vi "IntegerSynByteArray2.vi"(6 "Mode":T2(ring), 8 "Clock multiplier":u32=64, 9 "Local Oscillator (IF,f2)":u32, 10 "f (f1)":u32, 11 "Phase (degrees)":dbl=90.0) -> (1 "Actual ratios":T1 {"Clock" format="%_20p"; "F2" format="%_20p"; "F1" format="%_20p"; "Clock/F2" format="%_20g"; "Clock/F1" format="%_20g"}, 3 "output array":u8[](array[numeric]) format="%08b")   [LabVIEW 2015]
uses:
  Actual settings.ctl
panel:
  out "Clock":i32
  out "phase":u8 format="%08b"
  # "Heterodyne"
  # "IOtech      Synth           NatInstBrd\n              function          J7          P3                   P1\n              syn1 w clk       A0           3             P0.0  1\n              syn1 D7           A1           5             P0.1  3\n              syn2 w clk       A2           7             PO.2  5\n              syn2 D7           A3           9             PO.3  7\n              syn3 w clk       A4           4             PO.4  9\n              syn3 D7           A5           6             P0.5   11\n              syn1,2 FQ_UD  A6           8             PO.6   13\n              syn3 FQ_UD     A7          10            PO.7   15\n\n              Reset 1,2,3     B4          14             PFI3   23\n\n              SCLK              B0           13            PFI 0  17\n              SYNC              B1           15            PFI 1  19\n              DIN                B2           17             PFI 2  21"
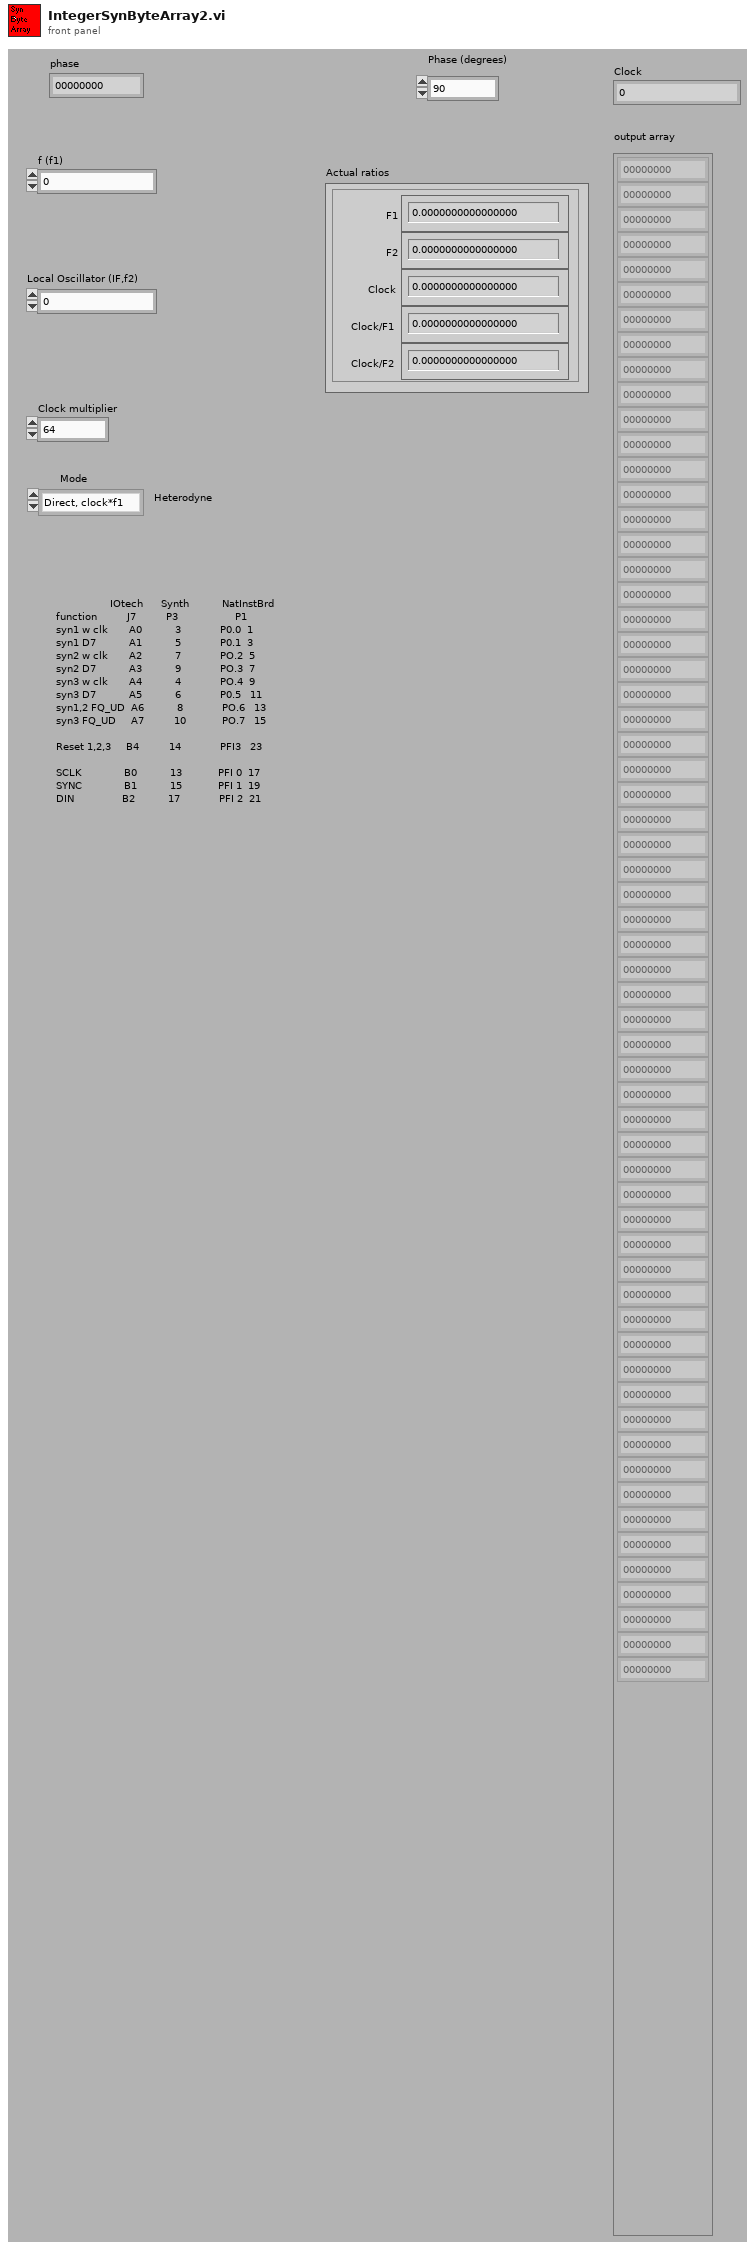
[diagram p1: front panel]
types:
  T1 = typedef "Actual settings.ctl" = cluster{"Clock/F1":ext, "Clock/F2":ext, "F1":ext, "F2":ext, "Clock":ext}
  T2 = enum16{"Direct, clock*f1", "Direct, clock*f2", "Heterodyne"}
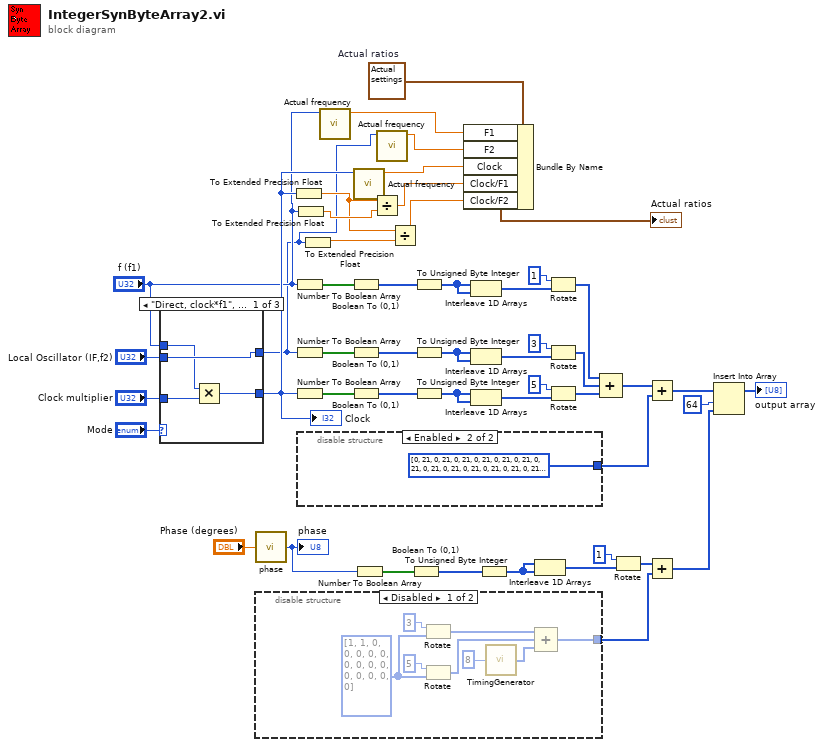
[diagram p0: block diagram]
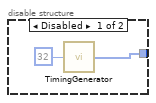
[diagram p2: hidden frame]
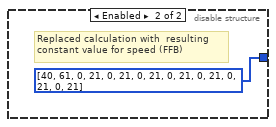
[diagram p3: hidden frame]
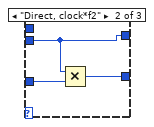
[diagram p4: hidden frame]
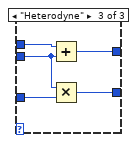
[diagram p5: hidden frame]
diagram:
  w7 = T1 {"Clock/F1"=64.0, "Clock/F2"=39.999998690327429603, "F1"=0.0, "F2"=0.0, "Clock"=0.0}  # Actual ratios
  n1 = case shown="\"Direct, clock*f1\", Default" "Mode" {
    tunnel: "Local Oscillator (IF,f2)" -> [w51 w54 w59]
    tunnel: [w53 w56 w61] -> w6
    tunnel: "Clock multiplier" -> [w52 w55 w60]
    tunnel: [w51 w54 w57] -> w2
    tunnel: "f (f1)" -> [w50 _ w58]
    frame "Direct, clock*f1", Default {
      n2 = Multiply(x=w50, y=w52) -> (x*y=w53:u32)
    }
    frame "Direct, clock*f2" {
      n3 = Multiply(x=w54, y=w55) -> (x*y=w56:u32)
    }
    frame "Heterodyne" {
      n4 = Add(x=w58, y=w59) -> (x+y=w57:u32)
      n5 = Multiply(x=w59, y=w60) -> (x*y=w61:u32)
    }
  }
  "Clock" <- w6
  n6 = call "phase.vi"("Phase"="Phase (degrees)") -> ("Phase Byte"=w24:u8)
  "phase" <- w24
  n7 = disable-structure shown="Disabled" {
    disable-tunnel: [w62 u8[] [40, 61, 0, 21, 0, 21, 0, 21, 0, 21, 0, 21, 0, 21, 0, 21] ("result")] -> w16
    frame Disabled {
      w64 = u8[] [1, 1, 0, 0, 0, 0, 0, 0, 0, 0, 0, 0, 0, 0, 0, 0] ("value")
      n8 = Rotate(1:w64, 2:i8 3) -> (0:w66:u8[])
      n9 = Rotate(1:w64, 2:i8 5) -> (0:w65:u8[])
      n10 = call "TimingGenerator.vi"("Clk String Lngth"=i8 8) -> ("TimingClock"=w63:u8[])
      n11 = Compound Arithmetic op=ADD(w66, w65, w63) -> (w62:u8[])
    }
    frame Enabled {
      # "Replaced calculation with  resulting \nconstant value for speed (FFB)"
    }
  }
  n12 = To Extended Precision Float(1:w6) -> (0:w11:ext)
  n13 = Number To Boolean Array(number="f (f1)") -> (Boolean array=w42:bool[])
  n14 = Number To Boolean Array(number=w2) -> (Boolean array=w47:bool[])
  n15 = Number To Boolean Array(number=w6) -> (Boolean array=w46:bool[])
  n16 = To Extended Precision Float(1:"f (f1)") -> (0:w13:ext)
  n17 = disable-structure shown="Enabled" {
    disable-tunnel: [w71 u8[] [0, 21, 0, 21, 0, 21, 0, 21, 0, 21, 0, 21, 0, 21, 0, 21, 0, 21, 0, 21, 0, 21, 0, 21, 0, 21, 0, 21, 0, 21, 0, 21, 0, 21, 0, 21, 0, 21, 0, 21, 0, 21, 0, 21, 0, 21, 0, 21, 0, 21, 0, 21, 0, 21, 0, 21, 0, 21, 0, 21, 0, 21, 0, 21] ("TimingClock")] -> w31
    frame Disabled {
      n18 = call "TimingGenerator.vi"("Clk String Lngth"=i8 32) -> ("TimingClock"=w71:u8[])
    }
    frame Enabled {
    }
  }
  n19 = To Extended Precision Float(1:w2) -> (0:w12:ext)
  n20 = call "Actual frequency.vi"("f-word"="f (f1)") -> ("Actual frequency, Hz"=w3:ext)  [unwired: 9 in, 1 out]
  n21 = Boolean To (0,1)(Boolean=w42) -> (0, 1=w41:i16[])
  n22 = Boolean To (0,1)(Boolean=w47) -> (0, 1=w45:i16[])
  n23 = Boolean To (0,1)(Boolean=w46) -> (0, 1=w44:i16[])
  n24 = call "Actual frequency.vi"("f-word"=w6) -> ("Actual frequency, Hz"=w5:ext)  [unwired: 9 in, 1 out]
  n25 = Number To Boolean Array(number=w24) -> (Boolean array=w27:bool[])
  n26 = Divide(x=w11, y=w13) -> (x/y=w10:ext)
  n27 = call "Actual frequency.vi"("f-word"=w2) -> ("Actual frequency, Hz"=w1:ext)  [unwired: 9 in, 1 out]
  n28 = Divide(x=w11, y=w12) -> (x/y=w9:ext)
  n29 = Boolean To (0,1)(Boolean=w27) -> (0, 1=w26:i16[])
  n30 = To Unsigned Byte Integer(number=w41) -> (unsigned 8bit integer=w30:u8[])
  n31 = To Unsigned Byte Integer(number=w45) -> (unsigned 8bit integer=w29:u8[])
  n32 = To Unsigned Byte Integer(number=w44) -> (unsigned 8bit integer=w28:u8[])
  n33 = Bundle By Name(cluster=w7, "F1"=w3, "F2"=w1, "Clock"=w5, "Clock/F1"=w10, "Clock/F2"=w9) -> (→"Actual ratios":T1)
  n34 = Interleave 1D Arrays(w30, w30) -> (w40:u8[])
  n35 = Interleave 1D Arrays(w29, w29) -> (w38:u8[])
  n36 = Interleave 1D Arrays(w28, w28) -> (w43:u8[])
  n37 = To Unsigned Byte Integer(number=w26) -> (unsigned 8bit integer=w23:u8[])
  n38 = Interleave 1D Arrays(w23, w23) -> (w25:u8[])
  n39 = Rotate(1:w40, 2:i8 1) -> (0:w33:u8[])
  n40 = Rotate(1:w38, 2:i8 3) -> (0:w34:u8[])
  n41 = Rotate(1:w43, 2:i8 5) -> (0:w35:u8[])
  n42 = Compound Arithmetic op=ADD(w33, w34, w35) -> (w32:u8[])
  n43 = Rotate(1:w25, 2:1) -> (0:w15:u8[])
  n44 = Add(x=w32, y=w31) -> (x+y=w19:u8[])
  n45 = Add(x=w15, y=w16) -> (x+y=w18:u8[])
  n46 = Insert Into Array(array=w19, index=64, new element=w18) -> (→"output array":u8[])
